vi "Startup.vi"(7 "App":refnum<class>, 8 "error in (no error)":errorcluster, 10 "Config":refnum<class>, 11 "Application in":refnum<class "Application.lvclass">) -> (0 "error out":errorcluster, 3 "Application out":refnum<class "Application.lvclass">)   [LabVIEW 2019, in "Application.lvclass"]
doc: "Developed by Kevin Thompson\nkevin@thompsonengineering.net\n\nCopyright 2018\nThompson Engineering, LLC"
uses:
  Application.lvclass
  Common/DataTypes/TD GetSet ActionSelect--enum.ctl
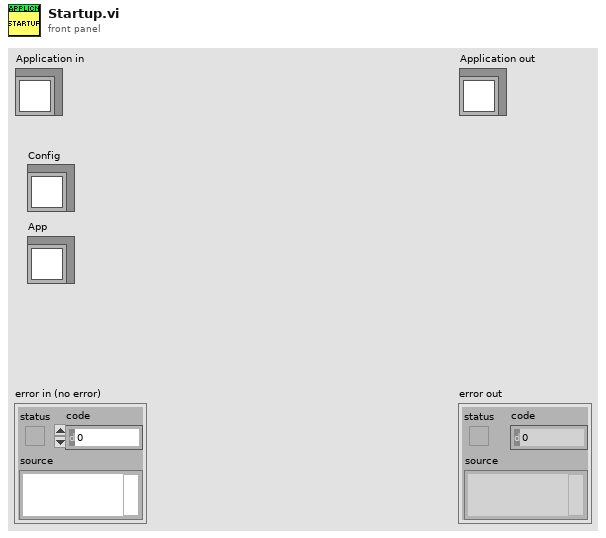
[diagram p1: front panel]
types:
  T1 = typedef "TD GetSet ActionSelect--enum.ctl" = enum16{"Init", "Get", "Set"}
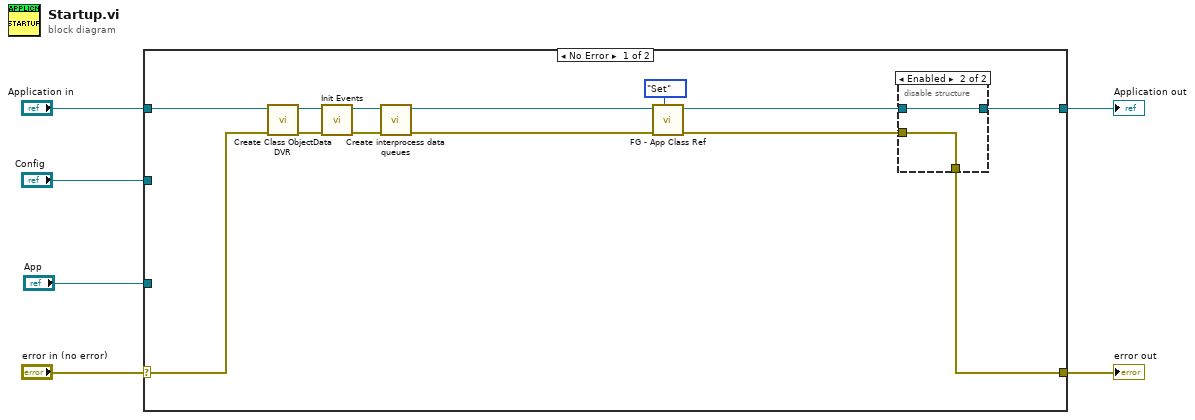
[diagram p0: block diagram]
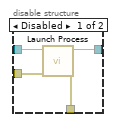
[diagram p2: hidden frame]
diagram:
  n1 = case shown="No Error" "error in (no error)" {
    selector: "error in (no error)" -> [w19 w27]
    tunnel: [w8 w27] -> w5
    tunnel: [w7 w26] -> w3
    tunnel: "Application in" -> [w18 w26]
    tunnel: "Config" -> [_ _]
    tunnel: "App" -> [_ _]
    frame No Error {
      n2 = call "Create Class ObjectData DVR.vi"("error in (no error)"=w19, "Application in"=w18) -> ("error out"=w16:errorcluster, "Application out"=w17:refnum<class "Application.lvclass">)  [unwired: 8 in]
      n3 = call "Init Events.vi"("error in (no error)"=w16, "Application in"=w17) -> ("error out"=w12:errorcluster, "Application out"=w11:refnum<class "Application.lvclass">)  [unwired: 8 in]
      n4 = call "Create interprocess data queues.vi"("error in (no error)"=w12, "Application in"=w11) -> ("error out"=w15:errorcluster, "Application out"=w14:refnum<class "Application.lvclass">)  [unwired: 6 in, 2 out]
      n5 = call "FG - App Class Ref.vi"("Application in"=w14, "error in (no error)"=w15, "action (Get)"=TD_GetSet_ActionSelect--enum."Set") -> ("Application out"=w10:refnum<class "Application.lvclass">, "error out"=w9:errorcluster)  [unwired: 6 in]
      n6 = disable-structure shown="Enabled" {
        disable-tunnel: w9 -> [w23 w24]
        disable-tunnel: w10 -> [w22 w25]
        disable-tunnel: [w21 w25] -> w7
        disable-tunnel: [w20 w24] -> w8
        frame Disabled {
          n7 = call "Launch Process.vi"("error in (no error)"=w23, "Application in"=w22) -> ("error out"=w20:errorcluster, "Application out"=w21:refnum<class "Application.lvclass">)  [unwired: 6 in, 2 out]
        }
        frame Enabled {
        }
      }
    }
    frame Error {
    }
  }
  "error out" <- w5
  "Application out" <- w3
